vi "ICM Read General Parameters.vi"(9 "Re-Init?":bool, 10 "ICM File In":path) -> (0 "error out":errorcluster, 1 "Parser":string, 2 "Bus":string, 3 "ICM General Parameters":T1 {"Start Time" format="%<%H:%M:%S>t"; "Date" format="%<%Y/%m/%d>T"; "Version" format="%.1g"}, 5 "Query":string)   [LabVIEW 2015]
doc: "ICM Read General Parameters.vi\n\nThis VI is used to read the General parameters from the ICM Configuration file.\n\nInstrument Communication Module Version 1.0\nAugust, 2017 Original Code Consulting David Thomson\n www.originalcode.com"
uses:
  Controls/ICM General Parameters.ctl
panel:
  # "The values for these\nparameters are generally\nset by the ICM system and\nneed not be edited directly."
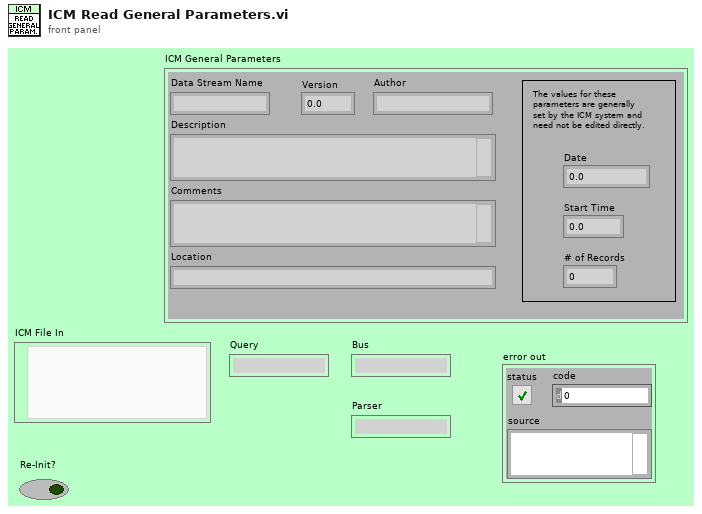
[diagram p1: front panel]
types:
  T1 = typedef "ICM General Parameters.ctl" = cluster{"Data Stream Name":string, "Version":sgl, "Author":string, "Description":string, "Comments":string, "Date":dbl, "Start Time":dbl, "Location":string, "# of Records":i32}
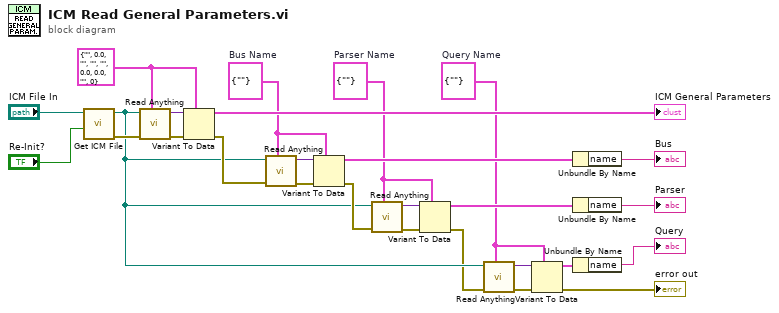
[diagram p0: block diagram]
diagram:
  w1 = cluster{"name":string} {"name"=""}  # Query Name
  w11 = cluster{"name":string} {"name"=""}  # Bus Name
  w12 = cluster{"name":string} {"name"=""}  # Parser Name
  w24 = T1 {"Data Stream Name"="", "Version"=0.0, "Author"="", "Description"="", "Comments"="", "Date"=0.0, "Start Time"=0.0, "Location"="", "# of Records"=0} ("ICM General Parameters")
  n1 = call "Get ICM File.vi"("Re-Init?"="Re-Init?", "ICM File In"="ICM File In") -> ("error out"=w27:errorcluster, "ICM File"=w5:path)  [unwired: 8 in]
  n2 = call "Read Anything.vi"("Type of Anything"=w24, "Error In"=w27, "Path (dialog)"=w5) -> ("Error Out"=w26:errorcluster, "Anything"=w23:variant)  [unwired: 6 in, 1 out]
  n3 = Variant To Data(error in=w26, type=w24, Variant=w23) -> (data=→"ICM General Parameters":T1, error out=w20:errorcluster)
  n4 = call "Read Anything.vi"("Type of Anything"=w11, "Error In"=w20, "Path (dialog)"=w5) -> ("Error Out"=w19:errorcluster, "Anything"=w18:variant)  [unwired: 6 in, 1 out]
  n5 = Variant To Data(error in=w19, type=w11, Variant=w18) -> (data=w17:cluster{"name":string}, error out=w14:errorcluster)
  n6 = call "Read Anything.vi"("Type of Anything"=w12, "Error In"=w14, "Path (dialog)"=w5) -> ("Error Out"=w15:errorcluster, "Anything"=w16:variant)  [unwired: 6 in, 1 out]
  n7 = Variant To Data(error in=w15, type=w12, Variant=w16) -> (data=w13:cluster{"name":string}, error out=w4:errorcluster)
  n8 = call "Read Anything.vi"("Type of Anything"=w1, "Error In"=w4, "Path (dialog)"=w5) -> ("Error Out"=w7:errorcluster, "Anything"=w6:variant)  [unwired: 6 in, 1 out]
  n9 = Variant To Data(error in=w7, type=w1, Variant=w6) -> (data=w8:cluster{"name":string}, error out=→"error out":errorcluster)
  n10 = Unbundle By Name(w17) -> ("name"=→"Bus":string)
  n11 = Unbundle By Name(w13) -> ("name"=→"Parser":string)
  n12 = Unbundle By Name(w8) -> ("name"=→"Query":string)
